vi "DisableCell.vi"(0 "DigitalCol in":refnum<class "DigitalCol.lvclass">, 5 "Cell Position":T1, 7 "Table Data in":string[][](array[string]), 9 "Table CtlRef In":refnum<vi>, 11 "error in (no error)":errorcluster) -> (4 "DigitalCol out":refnum<class "DigitalCol.lvclass">, 8 "Table Data out":string[][](array[string]), 10 "Table CtlRef Out":refnum<vi>, 15 "error out":errorcluster)   [LabVIEW 2013, in "DigitalCol.lvclass"]
uses:
  DigitalCol.lvclass
  <vilib>/Utility/miscctls.llb/LVRowAndColumnTypeDef.ctl
  Column/Column.lvclass/Column.ctl
  Column/Column.lvclass
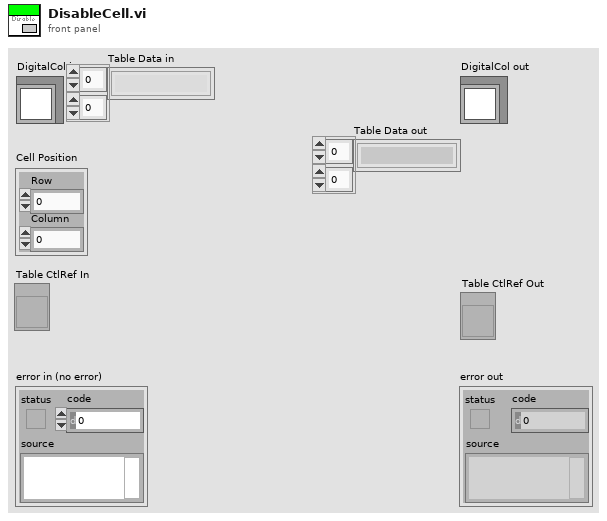
[diagram p1: front panel]
types:
  T1 = typedef "LVRowAndColumnTypeDef.ctl" = cluster{"Row":i32, "Column":i32}
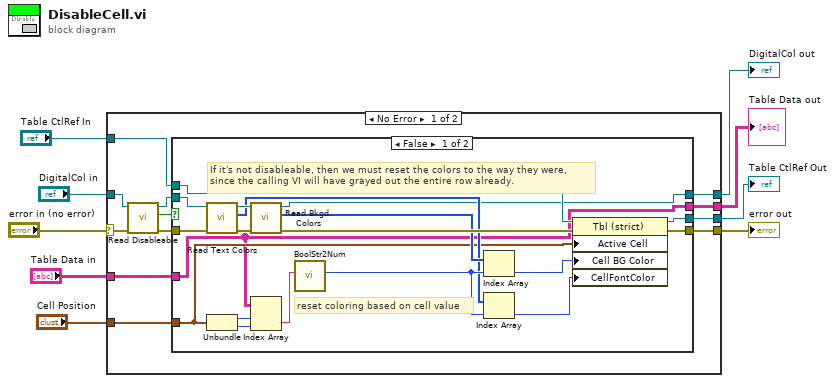
[diagram p0: block diagram]
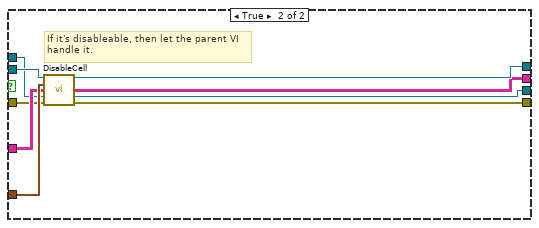
[diagram p2: hidden frame]
diagram:
  n1 = case shown="No Error" "error in (no error)" {
    selector: "error in (no error)" -> [w11 w53]
    tunnel: "DigitalCol in" -> [w14 w50]
    tunnel: [w21 w50] -> w8
    tunnel: "Cell Position" -> [w20 _]
    tunnel: "Table Data in" -> [w19 w51]
    tunnel: [w18 w51] -> w5
    tunnel: "Table CtlRef In" -> [w17 w52]
    tunnel: [w16 w52] -> w3
    tunnel: [w15 w53] -> w2
    frame No Error {
      n2 = call "Read Disableable.vi"("error in (no error)"=w11, "Column in"=w14) -> ("error out"=w10:errorcluster, "Disableable?"=w12:bool, "Column out"=w13:refnum<class "DigitalCol.lvclass">)  [unwired: 7 in]
      n3 = case shown="False" w12 {
        tunnel: w13 -> [w38 w49]
        tunnel: [w22 w48] -> w21
        tunnel: w20 -> [w26 w47]
        tunnel: w19 -> [w25 w46]
        tunnel: [w25 w45] -> w18
        tunnel: w17 -> [w30 w44]
        tunnel: [w24 w43] -> w16
        tunnel: [w23 w42] -> w15
        tunnel: w10 -> [w37 w41]
        frame False {
          # "reset coloring based on cell value"
          # "If it's not disableable, then we must reset the colors to the way they were,\nsince the calling VI will have grayed out the entire row already."
          n4 = call "Read Text Colors.vi"("error in (no error)"=w37, "Column in"=w38) -> ("error out"=w39:errorcluster, "Text Colors"=w27:u32[], "Column out"=w40:refnum<class "DigitalCol.lvclass">)  [unwired: 7 in]
          n5 = Unbundle(w26) -> ("Row"=w34:i32, "Column"=w33:i32)
          n6 = call "Read Bkgd. Colors.vi"("error in (no error)"=w39, "Column in"=w40) -> ("error out"=w29:errorcluster, "Bkgd. Colors"=w28:u32[], "Column out"=w22:refnum<class "DigitalCol.lvclass">)  [unwired: 7 in]
          n7 = Index Array(array=w25, index (row)=w34, index (col)=w33) -> (element=w32:string)
          n8 = call "BoolStr2Num.vi"("Boolean string"=w32) -> ("number"=w31:i32)  [unwired: 10 in]
          n9 = Index Array(array=w28, index=w31) -> (element=w36:u32)
          n10 = Index Array(array=w27, index=w31) -> (element=w35:u32)
          n11 = property class="Tbl (strict)"(reference=w30, error in=w29, "Active Cell"=w26, "Cell BG Color"=w36, "CellFontColor"=w35) -> (reference out=w24:refnum<vi>, error out=w23:errorcluster)
        }
        frame True {
          # "If it's disableable, then let the parent VI\nhandle it."
          n12 = call-parent "DisableCell.vi"("Column in"=w49, "Cell Position"=w47, "Table Data in"=w46, "Table CtlRef In"=w44, "error in (no error)"=w41) -> ("Column out"=w48:refnum<class "DigitalCol.lvclass">, "Table Data out"=w45:string[][], "Table CtlRef Out"=w43:refnum<vi>, "error out"=w42:errorcluster)  [unwired: 7 in]
        }
      }
    }
    frame Error {
    }
  }
  "error out" <- w2
  "DigitalCol out" <- w8
  "Table CtlRef Out" <- w3
  "Table Data out" <- w5
